vi "lpptx Sample.vi"() -> ()   [LabVIEW 2018]
uses:
  Size.ctl
  Position.ctl
  Font.ctl
  Slide Type.ctl
  lpptx.lvlib
panel:
  in  "Text":string="Hello world!"
  in  "Text formatting":T1={"Font"="Arial", "Size"=18.0, "Italic"=FALSE, "Bold"=FALSE, "Underline"=FALSE, "Color"=0}
  in  "Border":u32(colorbox)
  in  "Background":u32(colorbox)
  in  "Position":T2
  in  "Size":T3={"W"=500.0, "H"=100.0}
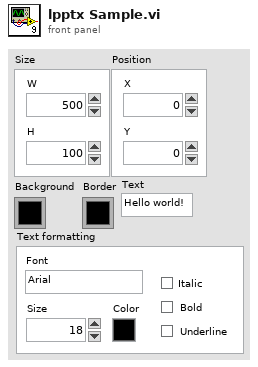
[diagram p1: front panel]
types:
  T1 = typedef "lpptx.lvlib/Font.ctl" = cluster{"Font":string, "Size":dbl, "Italic":bool, "Bold":bool, "Underline":bool, "Color":u32}
  T2 = typedef "Position.ctl" = cluster{"X":dbl, "Y":dbl}
  T3 = typedef "lpptx.lvlib/Size.ctl" = cluster{"W":dbl, "H":dbl}
  T4 = typedef "lpptx.lvlib/Slide Type.ctl" = i32
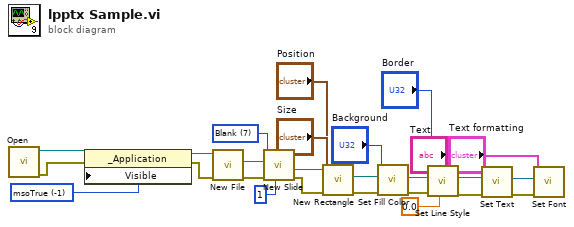
[diagram p0: block diagram]
diagram:
  w18 = T4 7 items=["Title Slide"=1, "Title and Content"=2, "Section Header"=3, "Two Content"=4, "Comparison"=5, "Title Only"=6, "Blank"=7] ("Type")
  w24 = -1 items=["msoTrue"=-1, "msoFalse"=0, "msoCTrue"=1, "msoTriStateToggle"=-3, "msoTriStateMixed"=-2] ("Visible")
  n1 = call "Open.vi"() -> ("error out"=w25:errorcluster, "Refnum"=w26:refnum<k7>)  [unwired: 10 in]
  n2 = property class="_Application"(reference=w26, error in=w25, "Visible"=w24) -> (reference out=w23:refnum<k7>, error out=w22:errorcluster)
  n3 = call "New File.vi"("error in (no error)"=w22, "Refnum"=w23) -> ("error out"=w21:errorcluster, "File refnum"=w20:refnum<k7>)  [unwired: 7 in, 1 out]
  n4 = call "New Slide.vi"("Offset"=1, "error in (no error)"=w21, "Type"=w18, "File refnum"=w20) -> ("error out"=w16:errorcluster, "Slide refnum out"=w17:refnum<k7>)  [unwired: 5 in, 1 out]
  n5 = call "New Rectangle.vi"("error in (no error)"=w16, "Position"="Position", "Size"="Size", "Slide refnum"=w17) -> ("error out"=w13:errorcluster, "Shape refnum out"=w12:refnum<k7>)  [unwired: 5 in, 1 out]
  n6 = call "Set Fill Color.vi"("error in (no error)"=w13, "Color"="Background", "Shape refnum"=w12) -> ("error out"=w10:errorcluster, "reference out"=w9:refnum<k7>)  [unwired: 7 in]
  n7 = call "Set Line Style.vi"("Weight (pt)"=sgl 0.0 ("Weight"), "error in (no error)"=w10, "Color"="Border", "Shape refnum"=w9) -> ("error out"=w6:errorcluster, "reference out"=w7:refnum<k7>)  [unwired: 6 in]
  n8 = call "Set Text.vi"("error in (no error)"=w6, "Text"="Text", "Shapre refnum"=w7) -> ("error out"=w5:errorcluster, "Shapre refnum out"=w4:refnum<k7>)  [unwired: 7 in]
  n9 = call "Set Font.vi"("error in (no error)"=w5, "Text formatting"="Text formatting", "Shape refnum"=w4) -> ()  [unwired: 7 in, 2 out]
